vi "Write Header Text.vi"(8 "error in (no error)":errorcluster, 10 "Header Text":string, 11 "Set Header Text in":refnum<class "Set Header Text.lvclass">) -> (0 "error out":errorcluster, 3 "Set Header Text out":refnum<class "Set Header Text.lvclass">)   [LabVIEW 2011, in "Set Header Text.lvclass"]
uses:
  Set Header Text.lvclass
  Set Header Text.lvclass/Set Header Text.ctl
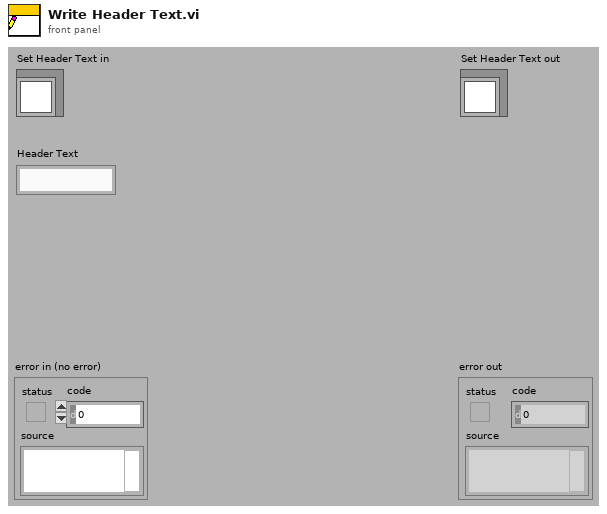
[diagram p1: front panel]
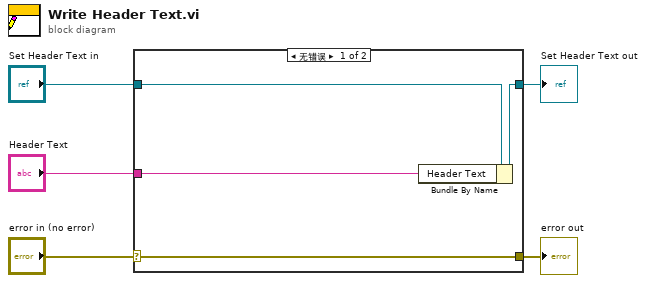
[diagram p0: block diagram]
diagram:
  n1 = case shown="无错误" "error in (no error)" {
    selector: "error in (no error)" -> [w9 w10]
    tunnel: [w9 w10] -> w4
    tunnel: [w7 w11] -> w2
    tunnel: "Set Header Text in" -> [w8 w11]
    tunnel: "Header Text" -> [w6 _]
    frame No Error {
      n2 = Bundle By Name(cluster=w8, "Header Text"=w6) -> (w7:refnum<class "Set Header Text.lvclass">)
    }
    frame Error {
    }
  }
  "error out" <- w4
  "Set Header Text out" <- w2
